vi "Untitled 2.vi"() -> ()   [LabVIEW 2012]
panel:
  out "selected path":path
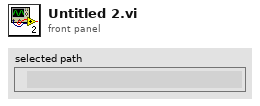
[diagram p1: front panel]
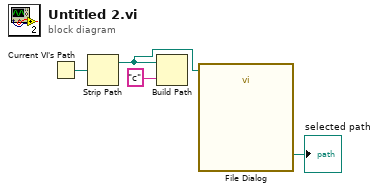
[diagram p0: block diagram]
diagram:
  n1 = Current VI's Path() -> (path=w2:path)
  n2 = Strip Path(path=w2) -> (stripped path=w1:path)  [unwired: 1 out]
  n3 = Build Path(base path=w1, name or relative path="c") -> ()  [unwired: 1 out]
  n4 = call "File Dialog"("start path"=w1) -> ("selected path"=→"selected path":path)  [unwired: 11 in, 3 out]
